vi "svx_Oct_Property Page.vi"(4 "# Plots Updated in":i32, 6 "Z Scale Graph Refnum":refnum<vi>, 7 "Main Graph":refnum<vi>, 8 "XY Scale Graph Refnum":refnum<vi>, 9 "Container Refnum":refnum<vi>, 10 "State in":T1={"X Scale Width %"=50.0, "Y Scale Height %"=50.0, "X-Axis Range"={"Minimum"=0.0, "Maximum"=10.0}, "Y-Axis Range"={"Minimum"=0.0, "Maximum"=10.0}, "Z-Axis Range"={"Minimum"=0.0, "Maximum"=10.0}, "Plot Color"=0, "Frame Color"=61212, "Background Color"=16252785, "Initial AutoScale Y"=TRUE, "AutoScale X"=2, "AutoScale Y"=2, "AutoScale Z"=2, "Plot Transparency"=FALSE, "X-Axis Name"="Frequency", "Y-Axis Name"="Amplitude", "Z-Axis Name"="", "X-Axis Scaling Factor"={"Offset"=0.0, "Multiplier"=1.0}, "Y-Axis Scaling Factor"={"Offset"=0.0, "Multiplier"=1.0}, "Z-Axis Scaling Factor"={"Offset"=0.0, "Multiplier"=1.0}, "X-Scale Visible"=TRUE, "Y-Scale Visible"=TRUE, "Z-Scale Visible"=TRUE, "X-Scale Label Visible"=TRUE, "Y-Scale Label Visible"=TRUE, "Z-Scale Label Visible"=TRUE, "X-Axis Range Scaled"={"Minimum"=0.0, "Maximum"=10.0}, "Y-Axis Range Scaled"={"Minimum"=0.0, "Maximum"=10.0}, "Z-Axis Range Scaled"={"Minimum"=0.0, "Maximum"=10.0}, "Rev Z Order"=FALSE, "X-Scale Format Str"="%#.4g", "Y-Scale Format Str"="%#.4g", "Z-Scale Format Str"="%#.4g", "Decor color"=12369084, "Scale Range Change"=refnum, "out of state queue"=refnum, "property nodes"=refnum} caption="State", 11 "Data In":T2={"z0"=0.0, "dz"=1.0, "Plots"=[]} {"Plots"."Y" format="%.2f"; "Plots"."X" format="%.2f"}) -> (0 "# Plots Updated out":i32, 1 "Cancel?":bool, 2 "State out":T1={"X Scale Width %"=50.0, "Y Scale Height %"=50.0, "X-Axis Range"={"Minimum"=0.0, "Maximum"=10.0}, "Y-Axis Range"={"Minimum"=0.0, "Maximum"=10.0}, "Z-Axis Range"={"Minimum"=0.0, "Maximum"=10.0}, "Plot Color"=0, "Frame Color"=61212, "Background Color"=16252785, "Initial AutoScale Y"=TRUE, "AutoScale X"=2, "AutoScale Y"=2, "AutoScale Z"=2, "Plot Transparency"=FALSE, "X-Axis Name"="Frequency", "Y-Axis Name"="Amplitude", "Z-Axis Name"="", "X-Axis Scaling Factor"={"Offset"=0.0, "Multiplier"=1.0}, "Y-Axis Scaling Factor"={"Offset"=0.0, "Multiplier"=1.0}, "Z-Axis Scaling Factor"={"Offset"=0.0, "Multiplier"=1.0}, "X-Scale Visible"=TRUE, "Y-Scale Visible"=TRUE, "Z-Scale Visible"=TRUE, "X-Scale Label Visible"=TRUE, "Y-Scale Label Visible"=TRUE, "Z-Scale Label Visible"=TRUE, "X-Axis Range Scaled"={"Minimum"=0.0, "Maximum"=10.0}, "Y-Axis Range Scaled"={"Minimum"=0.0, "Maximum"=10.0}, "Z-Axis Range Scaled"={"Minimum"=0.0, "Maximum"=10.0}, "Rev Z Order"=FALSE, "X-Scale Format Str"="%#.4g", "Y-Scale Format Str"="%#.4g", "Z-Scale Format Str"="%#.4g", "Decor color"=12369084, "Scale Range Change"=refnum, "out of state queue"=refnum, "property nodes"=refnum} caption="State")   [LabVIEW 2017, in "SVX Octave Waterfall Graph.xctl"]
uses:
  <vilib>/addons/_XControls/Octave Waterfall Graph/SVX Octave Waterfall Graph.xctl
  <vilib>/addons/_XControls/Octave Waterfall Graph/subVIs/svx_Oct_Waterfall Data.ctl
  <vilib>/addons/_XControls/Octave Waterfall Graph/subVIs/svx_Oct_Waterfall State.ctl
  <vilib>/addons/_XControls/Octave Waterfall Graph/subVIs/svx_Oct_Waterfall Property Page User Events.ctl
panel:
  in  "Help":bool
  in  "Cancel":bool
  in  "OK":bool
  in  "Tab Control":T3(tab)
  in  "Reverse Order":bool
  in  "Plot Transparency":bool
  in  "Background color":u32(colorbox)
  in  "Frame color":u32(colorbox)
  in  "Plot color":u32(colorbox)
  in  "Enable State":T4(radio)
  in  "Caption":string
  in  "Label":string
  in  "Caption Visible?":bool
  in  "Label Visible?":bool
  in  "trailing zeros":bool
  in  "Digits":u8=1
  in  "Precision Type":u16(ring) caption="Precision type" items=["Digits of precision", "Significant digits"]
  in  "Type":i32(listbox)
  in  "FP Axis":enum16{"X-Axis", "Y-Axis", "Z-Axis"}(ring)
  in  "Scaling Factors - Multiplier":dbl caption="Multiplier"
  in  "Scaling Factors - Offset":dbl caption="Offset"
  in  "Range Maximum":dbl caption="Maximum"
  in  "Range Minimum":dbl caption="Minimum"
  in  "Autoscale":bool
  in  "Show Scale":bool
  in  "Show Scale label":bool
  in  "Scale Name":string caption="Name"
  in  "Scale Axis":enum16{"X-Axis", "Y-Axis", "Z-Axis"}(ring)
  in  "Tip strip":string
  in  "Description":string
  # "Label"
  # "Caption"
  # "Enabled State"
  # "Color Scheme"
  # "Scaling factors"
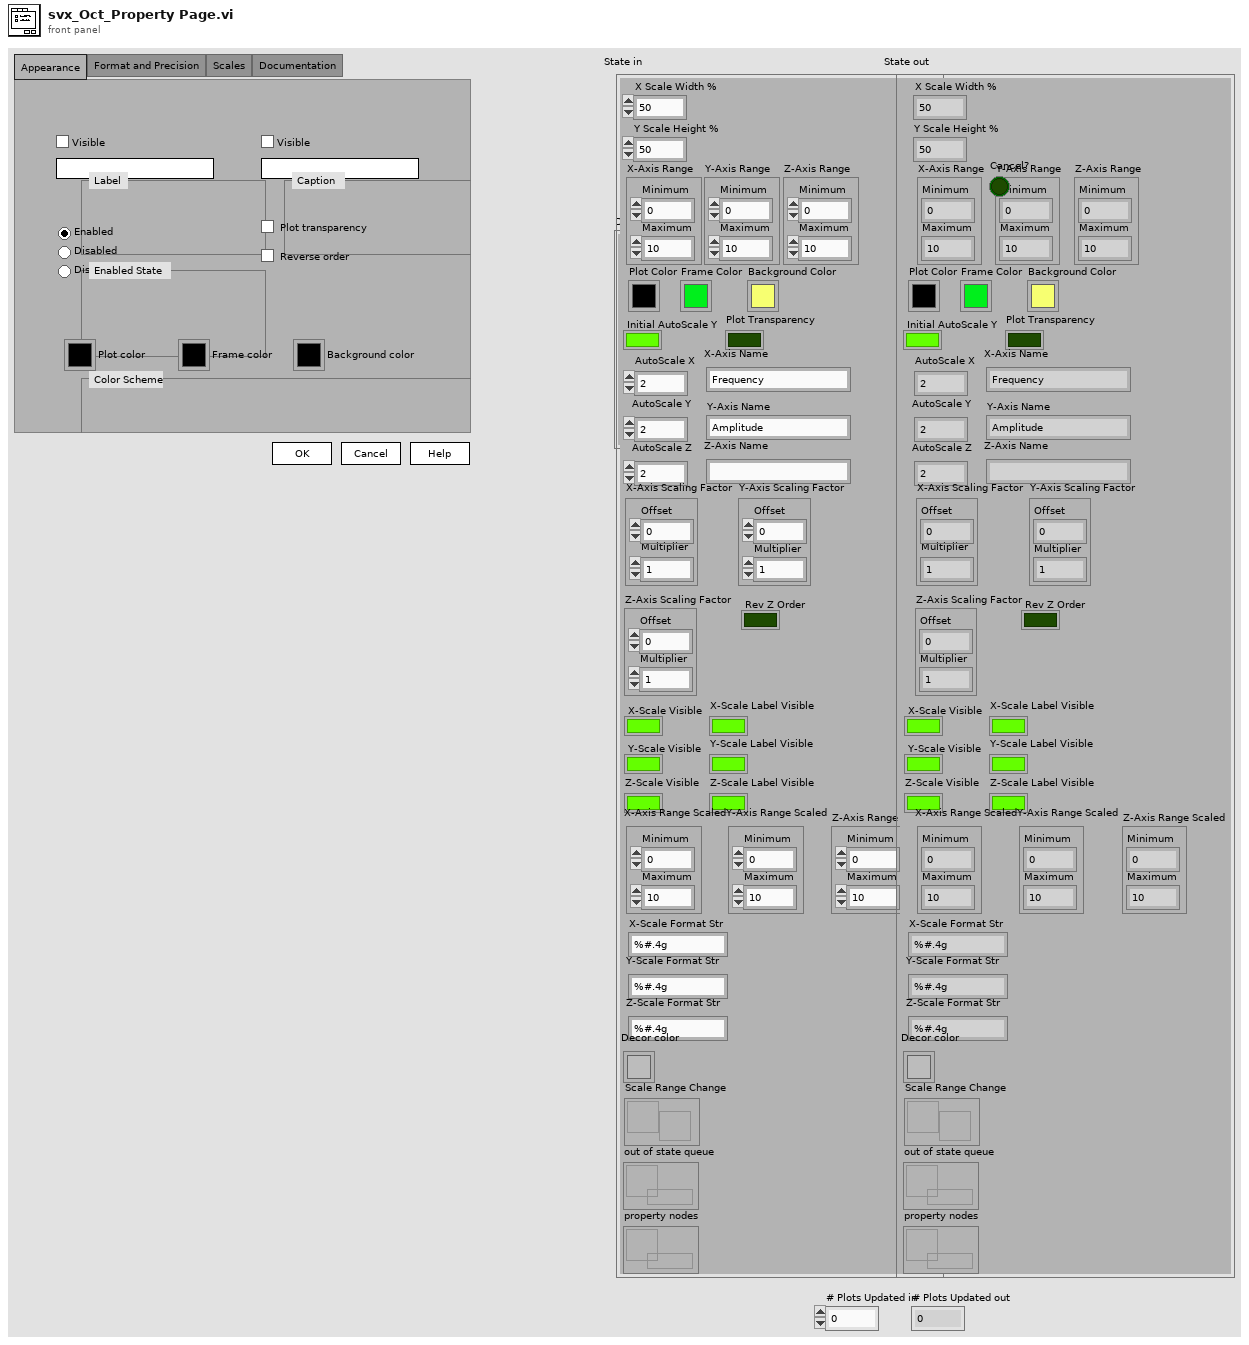
[diagram p1: front panel]
types:
  T1 = typedef "SVX Octave Waterfall Graph.xctl/svx_Oct_Waterfall State.ctl" = cluster{"X Scale Width %":dbl, "Y Scale Height %":dbl, "X-Axis Range":cluster{"Minimum":dbl, "Maximum":dbl}, "Y-Axis Range":cluster{"Minimum":dbl, "Maximum":dbl}, "Z-Axis Range":cluster{"Minimum":dbl, "Maximum":dbl}, "Plot Color":u32, "Frame Color":u32, "Background Color":u32, "Initial AutoScale Y":bool, "AutoScale X":u8, "AutoScale Y":u8, "AutoScale Z":u8, "Plot Transparency":bool, "X-Axis Name":string, "Y-Axis Name":string, "Z-Axis Name":string, "X-Axis Scaling Factor":cluster{"Offset":dbl, "Multiplier":dbl}, "Y-Axis Scaling Factor":cluster{"Offset":dbl, "Multiplier":dbl}, "Z-Axis Scaling Factor":cluster{"Offset":dbl, "Multiplier":dbl}, "X-Scale Visible":bool, "Y-Scale Visible":bool, "Z-Scale Visible":bool, "X-Scale Label Visible":bool, "Y-Scale Label Visible":bool, "Z-Scale Label Visible":bool, "X-Axis Range Scaled":cluster{"Minimum":dbl, "Maximum":dbl}, "Y-Axis Range Scaled":cluster{"Minimum":dbl, "Maximum":dbl}, "Z-Axis Range Scaled":cluster{"Minimum":dbl, "Maximum":dbl}, "Rev Z Order":bool, "X-Scale Format Str":string, "Y-Scale Format Str":string, "Z-Scale Format Str":string, "Decor color":u32, "Scale Range Change":refnum<user-event>, "out of state queue":refnum<queue>, "property nodes":refnum<queue>}
  T2 = typedef "SVX Octave Waterfall Graph.xctl/svx_Oct_Waterfall Data.ctl" = cluster{"z0":dbl, "dz":dbl, "Plots":cluster{"X":dbl[], "Y":dbl[]}[]}
  T3 = enum32{"Appearance", "Format and Precision", "Scales", "Documentation"}
  T4 = enum32{"Enabled", "Disabled", "Disabled & grayed"}
  T5 = typedef "SVX Octave Waterfall Graph.xctl/svx_Oct_Waterfall Property Page User Events.ctl" = enum16{"Redraw Frame", "Update Graph", "Exit"}
  T6 = cluster{"Container Changed":bool, "Scales Changed":bool, "Waveform Changed":bool}
  T7 = cluster{"Label.Text":string, "Label.Visible":bool, "Caption.Text":string, "Caption.Visible":bool, "Disabled":u8, "Desc":string, "TipStrip":string}
  T8 = cluster{"Width":u16, "Style":enum32{"Solid", "Dash", "Dot", "DashDot", "DashDotDot"}}
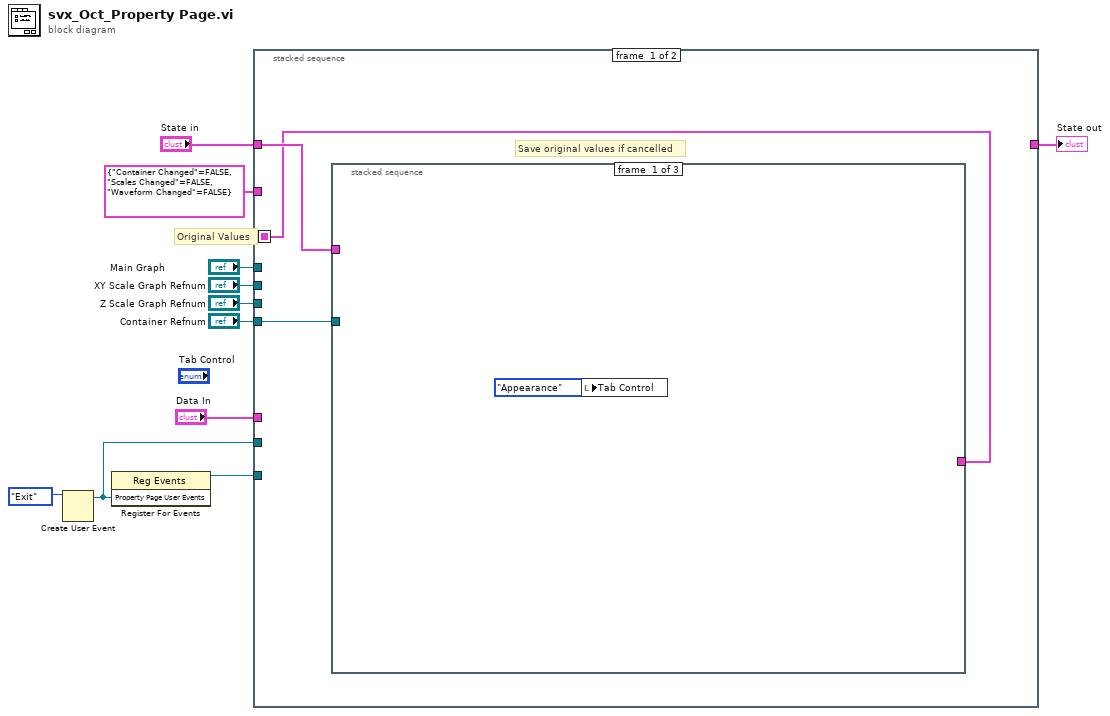
[diagram p0: block diagram]
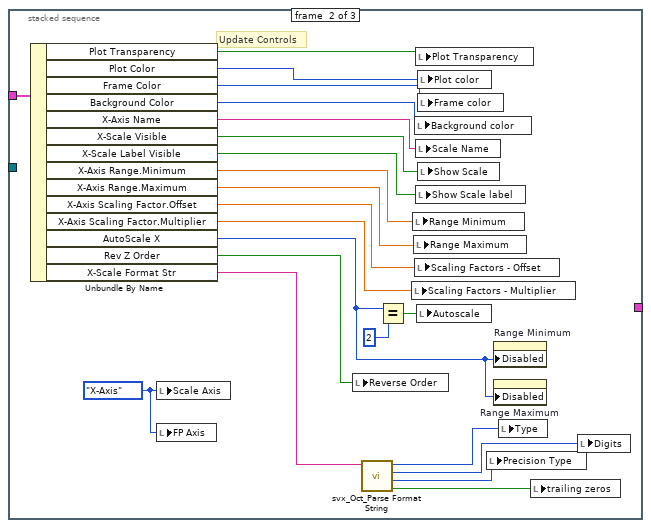
[diagram p2: hidden frame]
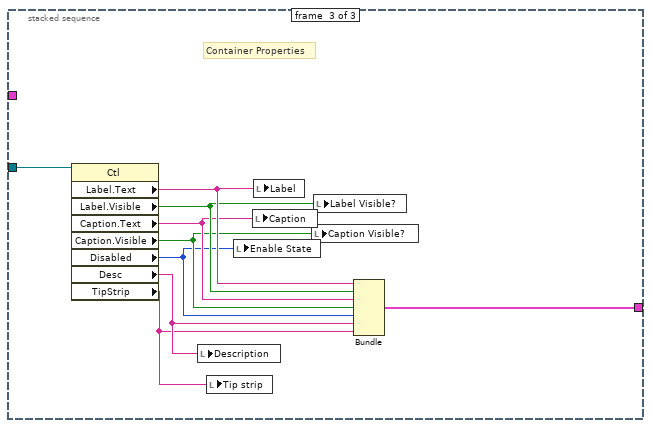
[diagram p3: hidden frame]
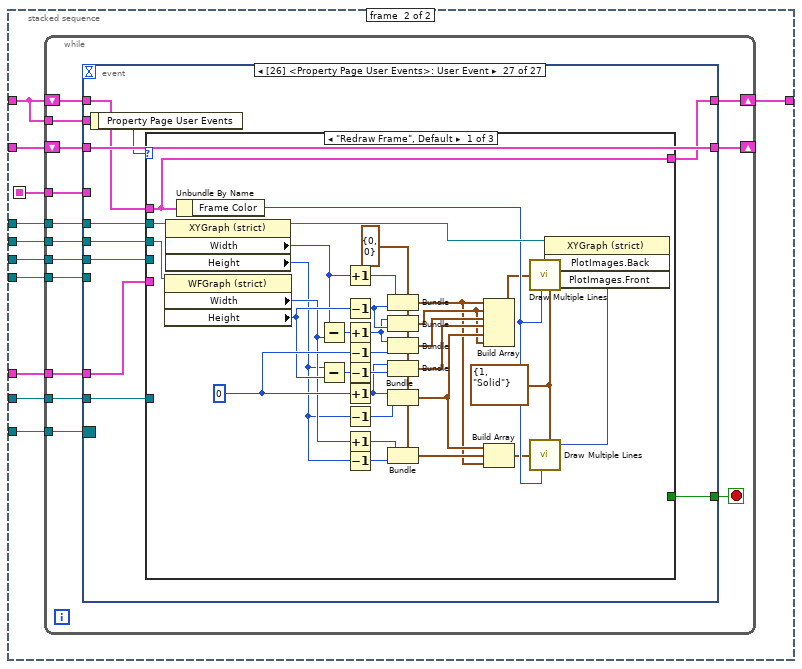
[diagram p4: hidden frame]
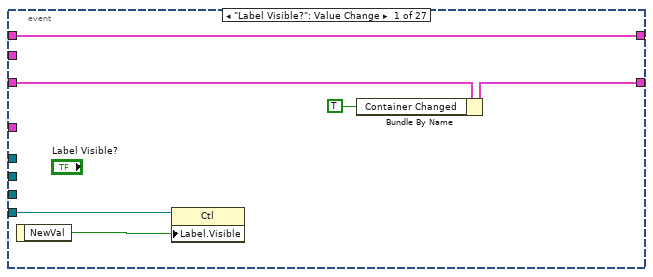
[diagram p5: hidden frame]
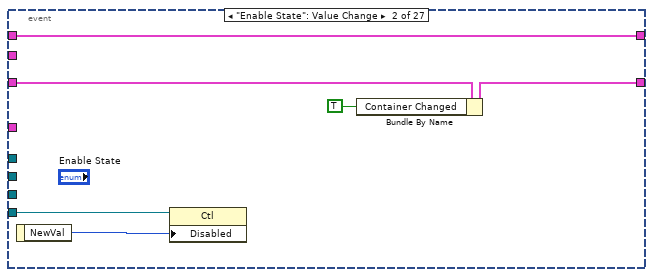
[diagram p6: hidden frame]
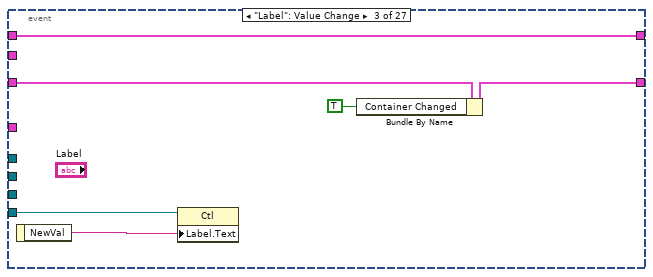
[diagram p7: hidden frame]
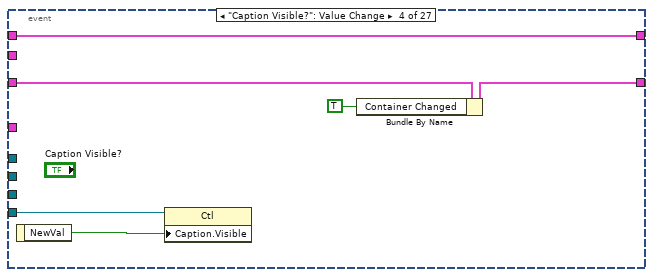
[diagram p8: hidden frame]
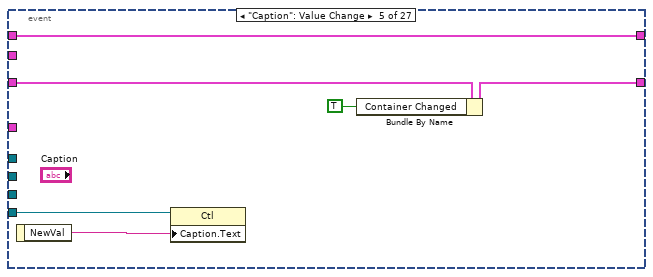
[diagram p9: hidden frame]
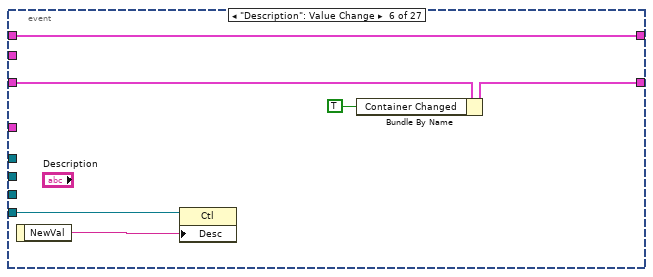
[diagram p10: hidden frame]
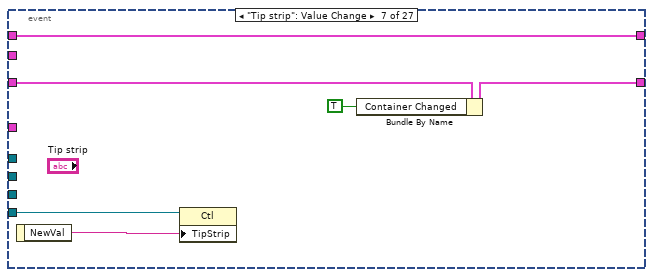
[diagram p11: hidden frame]
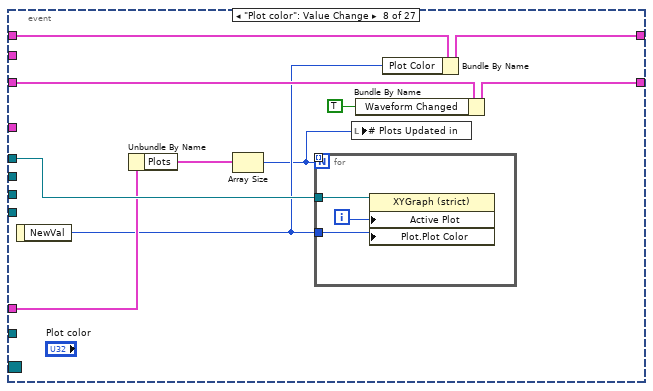
[diagram p12: hidden frame]
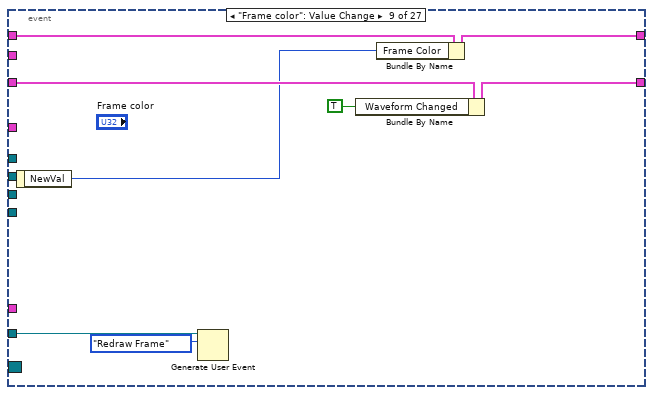
[diagram p13: hidden frame]
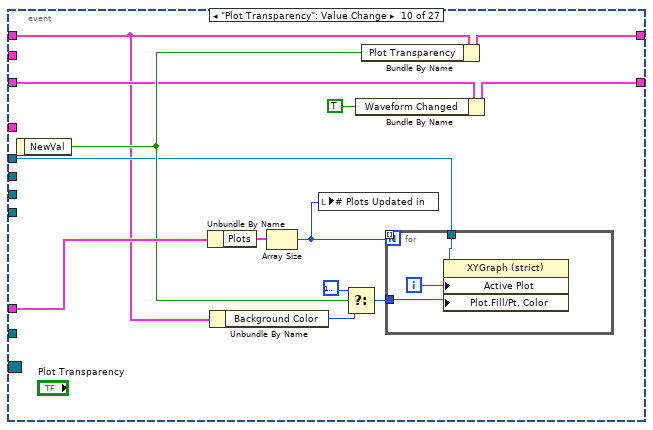
[diagram p14: hidden frame]
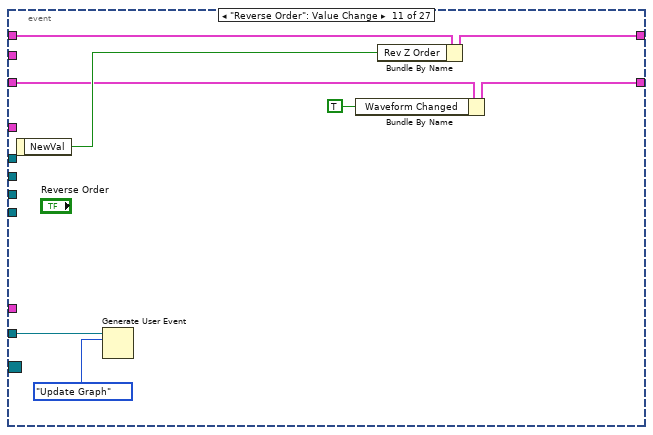
[diagram p15: hidden frame]
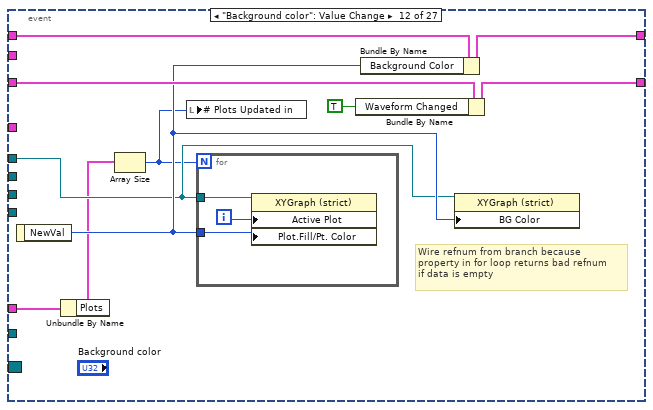
[diagram p16: hidden frame]
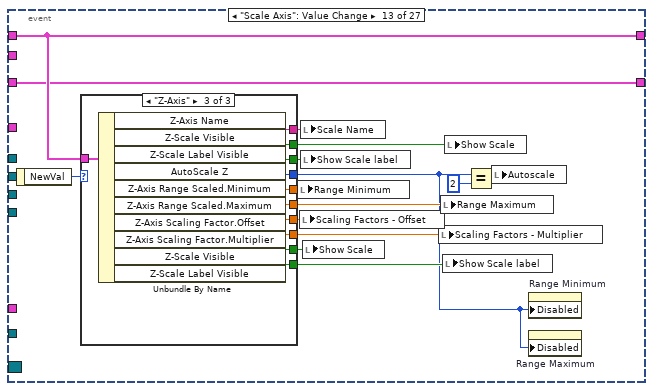
[diagram p17: hidden frame]
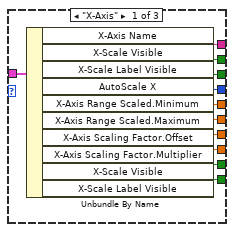
[diagram p18: hidden frame]
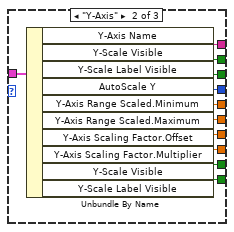
[diagram p19: hidden frame]
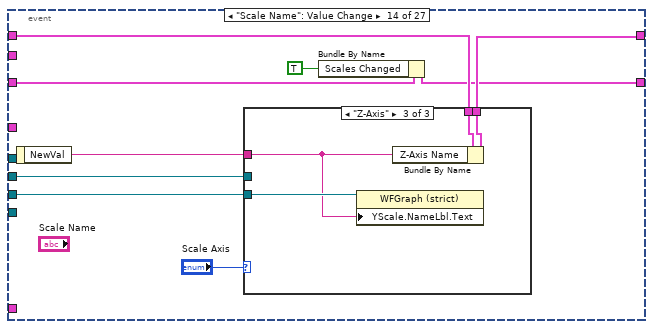
[diagram p20: hidden frame]
diagram:
  # "Original Values"
  n1 = Create User Event(user event datatype=svx_Oct_Waterfall_Property_Page_User_Events."Exit" ("Property Page User Events")) -> (user event=w1:refnum<user-event>)  [unwired: 1 in, 1 out]
  n2 = register-events(w1) -> (reference out=w3:refnum<event-registration>)  [unwired: 2 in, 1 out]
  n3 = stacked-sequence {
    seq-local: [w12 _] -> [_ w50]
    tunnel: T6 {"Container Changed"=FALSE, "Scales Changed"=FALSE, "Waveform Changed"=FALSE} -> [_ w57]
    tunnel: "Main Graph" -> [_ w56]
    tunnel: "XY Scale Graph Refnum" -> [_ w55]
    tunnel: "Z Scale Graph Refnum" -> [_ w54]
    tunnel: "Container Refnum" -> [w14 w53]
    tunnel: "State in" -> [w13 w51]
    tunnel: [_ w52] -> w5
    tunnel: "Data In" -> [_ w49]
    tunnel: w3 -> [_ w48]
    tunnel: w1 -> [_ w47]
    frame #0 {
      # "Save original values if cancelled"
      n4 = stacked-sequence {
        tunnel: w14 -> [_ _ w46]
        tunnel: [_ _ w45] -> w12
        tunnel: w13 -> [_ w37 _]
        frame #0 {
          n5 = local write "Tab Control"(T3."Appearance" ("Tab Control")) -> ()
        }
        frame #1 {
          w16 = enum16{"X-Axis", "Y-Axis", "Z-Axis"}."X-Axis" ("Axis")
          # "Update Controls"
          n6 = Unbundle By Name(w37) -> ("Plot Transparency"=w26:bool, "Plot Color"=w36:u32, "Frame Color"=w35:u32, "Background Color"=w34:u32, "X-Axis Name"=w33:string, "X-Scale Visible"=w32:bool, "X-Scale Label Visible"=w31:bool, "X-Axis Range.Minimum"=w30:dbl, "X-Axis Range.Maximum"=w29:dbl, "X-Axis Scaling Factor.Offset"=w28:dbl, "X-Axis Scaling Factor.Multiplier"=w27:dbl, "AutoScale X"=w25:u8, "Rev Z Order"=w22:bool, "X-Scale Format Str"=w21:string)
          n7 = local write "Scale Axis"(w16) -> ()
          n8 = local write "FP Axis"(w16) -> ()
          n9 = local write "Reverse Order"(w22) -> ()
          n10 = call <vilib>:"svx_Oct_Parse Format String.vi"("Format string"=w21) -> ("trailing zeros"=w17:bool, "Precision Type"=w18:u16, "Digits"=w19:u8, "Type"=w20:i32)  [unwired: 6 in, 1 out]
          n11 = Equal?(x=w25, y=u8 2) -> (x = y?=w23:bool)
          n12 = local write "Scaling Factors - Multiplier"(w27) -> ()
          n13 = local write "Range Minimum"(w30) -> ()
          n14 = local write "Range Maximum"(w29) -> ()
          n15 = local write "Background color"(w34) -> ()
          n16 = local write "Scaling Factors - Offset"(w28) -> ()
          n17 = local write "Plot Transparency"(w26) -> ()
          n18 = local write "Scale Name"(w33) -> ()
          n19 = local write "Show Scale label"(w31) -> ()
          n20 = local write "Autoscale"(w23) -> ()
          n21 = local write "Plot color"(w36) -> ()
          n22 = local write "Frame color"(w35) -> ()
          n23 = local write "Show Scale"(w32) -> ()
          n24 = local write "Precision Type"(w18) -> ()
          n25 = property on="Range Minimum" class="DigNum (strict)"("Disabled"=w25) -> ()  [unwired: 2 in, 2 out]
          n26 = property on="Range Maximum" class="DigNum (strict)"("Disabled"=w25) -> ()  [unwired: 2 in, 2 out]
          n27 = local write "Type"(w20) -> ()
          n28 = local write "trailing zeros"(w17) -> ()
          n29 = local write "Digits"(w19) -> ()
        }
        frame #2 {
          # "Container Properties"
          n30 = property class="Ctl"(reference=w46) -> ("Label.Text"=w44:string, "Label.Visible"=w43:bool, "Caption.Text"=w42:string, "Caption.Visible"=w41:bool, "Disabled"=w40:u8, "Desc"=w39:string, "TipStrip"=w38:string)  [unwired: 1 in, 2 out]
          n31 = local write "Description"(w39) -> ()
          n32 = local write "Tip strip"(w38) -> ()
          n33 = local write "Enable State"(w40) -> ()
          n34 = local write "Caption"(w42) -> ()
          n35 = local write "Label"(w44) -> ()
          n36 = local write "Caption Visible?"(w41) -> ()
          n37 = local write "Label Visible?"(w43) -> ()
          n38 = Bundle("Label.Text"=w44, "Label.Visible"=w43, "Caption.Text"=w42, "Caption.Visible"=w41, "Disabled"=w40, "Desc"=w39, "TipStrip"=w38) -> (w45:T7)  [unwired: 1 in]
        }
      }
    }
    frame #1 {
      n39 = while {
        shift-right: [w69] -> _
        shift-left: w57 -> [w70]
        tunnel: w56 -> [w68]
        tunnel: w55 -> [w67]
        tunnel: w54 -> [w66]
        tunnel: w53 -> [w65]
        shift-right: [w63] -> w52
        shift-left: w51 -> [w64]
        tunnel: w51 -> [w62]
        tunnel: w50 -> [w61]
        tunnel: w49 -> [w60]
        tunnel: w48 -> [w59]
        tunnel: w47 -> [w58]
        stop <- w71 stop-if-true
        n40 = event shown="[26] <Property Page User Events>: User Event" {
          selector: w59 -> [_ _ _ _ _ _ _ _ _ _ _ _ _ _ _ _ _ _ _ _ _ _ _ _ _ _ _]
          dyn-events: _ -> [_ _ _ _ _ _ _ _ _ _ _ _ _ _ _ _ _ _ _ _ _ _ _ _ _ _ _]
          timeout: _ -> [_ _ _ _ _ _ _ _ _ _ _ _ _ _ _ _ _ _ _ _ _ _ _ _ _ _ _]
          tunnel: [_ _ _ _ _ _ _ _ _ _ _ _ _ _ _ _ _ _ _ _ _ _ _ w547 _ _ w641] -> w71
          tunnel: w70 -> [w77 w83 w89 w95 w101 w107 w113 w123 w135 w141 w156 w170 w179 w223 w245 w266 w287 w338 w394 w442 w493 w514 w531 w551 w560 w630 w643]
          tunnel: [w76 w82 w88 w94 w100 w106 w112 w122 w134 w148 w160 w169 w179 w222 w244 w265 w286 w337 w393 w441 w492 w514 w530 w551 w560 w630 w643] -> w69
          tunnel: w68 -> [_ _ _ _ _ _ _ w120 _ w139 _ w163 _ _ _ _ _ _ w398 w446 _ _ _ _ w555 _ w640]
          tunnel: w67 -> [_ _ _ _ _ _ _ _ _ _ _ _ _ w226 w248 w269 w293 w344 w401 w449 _ _ w527 _ w553 _ w639]
          tunnel: w66 -> [_ _ _ _ _ _ _ _ _ _ _ _ _ w225 w247 w268 w292 w343 w400 w448 _ _ w526 _ w552 _ w635]
          tunnel: w65 -> [w74 w80 w86 w92 w98 w104 w110 _ _ _ _ _ _ _ _ _ _ _ _ _ _ _ _ _ w559 _ _]
          tunnel: w64 -> [w72 w78 w84 w90 w96 w102 w108 w119 w132 w138 w155 w167 w187 w230 w251 w272 w296 w347 w404 w452 w498 w513 w534 w550 _ w629 w637]
          tunnel: [w72 w78 w84 w90 w96 w102 w108 w118 w131 w146 w158 w166 w187 w229 w250 w271 w295 w346 w403 w451 w497 w513 w533 w550 w557 w629 w634] -> w63
          tunnel: w62 -> [_ _ _ _ _ _ _ _ _ _ _ _ _ _ _ _ _ _ _ _ _ _ _ _ w557 _ _]
          tunnel: w61 -> [_ _ _ _ _ _ _ _ _ _ _ _ _ _ _ _ _ _ _ _ _ _ _ _ w554 _ _]
          tunnel: w60 -> [_ _ _ _ _ _ _ w117 _ w144 _ w165 _ _ _ _ _ _ _ _ _ _ _ _ w556 _ w638]
          tunnel: w58 -> [_ _ _ _ _ _ _ _ w129 _ w153 _ _ _ _ _ w285 w336 w397 w445 w496 _ _ w548 w558 _ w636]
          event "Label Visible?": Value Change {
            n41 = event-data() -> ("NewVal"=w73:bool)  [unwired: 1 in]
            n42 = property class="Ctl"(reference=w74, "Label.Visible"=w73) -> ()  [unwired: 1 in, 2 out]
            n43 = Bundle By Name(cluster=w77, "Container Changed"=TRUE) -> (w76:T6)
          }
          event "Enable State": Value Change {
            n44 = event-data() -> ("NewVal"=w79:T4)  [unwired: 1 in]
            n45 = property class="Ctl"(reference=w80, "Disabled"=w79) -> ()  [unwired: 1 in, 2 out]
            n46 = Bundle By Name(cluster=w83, "Container Changed"=TRUE) -> (w82:T6)
          }
          event "Label": Value Change {
            n47 = event-data() -> ("NewVal"=w85:string)  [unwired: 1 in]
            n48 = property class="Ctl"(reference=w86, "Label.Text"=w85) -> ()  [unwired: 1 in, 2 out]
            n49 = Bundle By Name(cluster=w89, "Container Changed"=TRUE) -> (w88:T6)
          }
          event "Caption Visible?": Value Change {
            n50 = event-data() -> ("NewVal"=w91:bool)  [unwired: 1 in]
            n51 = property class="Ctl"(reference=w92, "Caption.Visible"=w91) -> ()  [unwired: 1 in, 2 out]
            n52 = Bundle By Name(cluster=w95, "Container Changed"=TRUE) -> (w94:T6)
          }
          event "Caption": Value Change {
            n53 = event-data() -> ("NewVal"=w97:string)  [unwired: 1 in]
            n54 = property class="Ctl"(reference=w98, "Caption.Text"=w97) -> ()  [unwired: 1 in, 2 out]
            n55 = Bundle By Name(cluster=w101, "Container Changed"=TRUE) -> (w100:T6)
          }
          event "Description": Value Change {
            n56 = event-data() -> ("NewVal"=w103:string)  [unwired: 1 in]
            n57 = property class="Ctl"(reference=w104, "Desc"=w103) -> ()  [unwired: 1 in, 2 out]
            n58 = Bundle By Name(cluster=w107, "Container Changed"=TRUE) -> (w106:T6)
          }
          event "Tip strip": Value Change {
            n59 = event-data() -> ("NewVal"=w109:string)  [unwired: 1 in]
            n60 = property class="Ctl"(reference=w110, "TipStrip"=w109) -> ()  [unwired: 1 in, 2 out]
            n61 = Bundle By Name(cluster=w113, "Container Changed"=TRUE) -> (w112:T6)
          }
          event "Plot color": Value Change {
            n62 = event-data() -> ("NewVal"=w116:u32)  [unwired: 1 in]
            n63 = Unbundle By Name(w117) -> ("Plots"=w115:cluster{"X":dbl[], "Y":dbl[]}[])
            n64 = Array Size(array=w115) -> (size(s)=w114:i32)
            n65 = for {
              N: w114 -> [w124]
              tunnel: w116 -> [w126]
              tunnel: w120 -> [w127]
              tunnel: [w124] -> _ mode=indexing
              i -> [w125]
              n66 = property class="XYGraph (strict)"(reference=w127, "Active Plot"=w125, "Plot.Plot Color"=w126) -> ()  [unwired: 1 in, 2 out]
            }
            n67 = local write "# Plots Updated in"(w114) -> ()
            n68 = Bundle By Name(cluster=w123, "Waveform Changed"=TRUE ("Container Changed")) -> (w122:T6)
            n69 = Bundle By Name(cluster=w119, "Plot Color"=w116) -> (w118:T1)
          }
          event "Frame color": Value Change {
            n70 = event-data() -> ("NewVal"=w130:u32)  [unwired: 1 in]
            n71 = Generate User Event(user event=w129, event data cluster=svx_Oct_Waterfall_Property_Page_User_Events."Redraw Frame" ("Property Page User Events")) -> ()  [unwired: 2 in, 2 out]
            n72 = Bundle By Name(cluster=w135, "Waveform Changed"=TRUE ("Container Changed")) -> (w134:T6)
            n73 = Bundle By Name(cluster=w132, "Frame Color"=w130) -> (w131:T1)
          }
          event "Plot Transparency": Value Change {
            n74 = event-data() -> ("NewVal"=w143:bool)  [unwired: 1 in]
            n75 = Unbundle By Name(w144) -> ("Plots"=w137:cluster{"X":dbl[], "Y":dbl[]}[])
            n76 = Unbundle By Name(w138) -> ("Background Color"=w140:u32)
            n77 = Array Size(array=w137) -> (size(s)=w136:i32)
            n78 = local write "# Plots Updated in"(w136) -> ()
            n79 = Select(t=u32 16777216, s=w143, f=w140) -> (s? t:f=w145:u32)
            n80 = Bundle By Name(cluster=w141, "Waveform Changed"=TRUE) -> (w148:T6)
            n81 = Bundle By Name(cluster=w138, "Plot Transparency"=w143) -> (w146:T1)
            n82 = for {
              N: w136 -> [w149]
              tunnel: w145 -> [w151]
              tunnel: w139 -> [w150]
              tunnel: [w149] -> _ mode=indexing
              i -> [w152]
              n83 = property on="Property Node" class="XYGraph (strict)"(reference=w150, "Active Plot"=w152, "Plot.Fill/Pt. Color"=w151) -> ()  [unwired: 1 in, 2 out]
            }
          }
          event "Reverse Order": Value Change {
            n84 = event-data() -> ("NewVal"=w157:bool)  [unwired: 1 in]
            n85 = Generate User Event(user event=w153, event data cluster=svx_Oct_Waterfall_Property_Page_User_Events."Update Graph" ("event data")) -> ()  [unwired: 2 in, 2 out]
            n86 = Bundle By Name(cluster=w156, "Waveform Changed"=TRUE) -> (w160:T6)
            n87 = Bundle By Name(cluster=w155, "Rev Z Order"=w157) -> (w158:T1)
          }
          event "Background color": Value Change {
            # "Wire refnum from branch because\nproperty in for loop returns bad refnum\nif data is empty"
            n88 = event-data() -> ("NewVal"=w164:u32)  [unwired: 1 in]
            n89 = Unbundle By Name(w165) -> ("Plots"=w162:cluster{"X":dbl[], "Y":dbl[]}[])
            n90 = Array Size(array=w162) -> (size(s)=w161:i32)
            n91 = local write "# Plots Updated in"(w161) -> ()
            n92 = for {
              N: w161 -> [_]
              tunnel: w164 -> [w172]
              tunnel: w163 -> [w173]
              i -> [w171]
              n93 = property class="XYGraph (strict)"(reference=w173, "Active Plot"=w171, "Plot.Fill/Pt. Color"=w172) -> ()  [unwired: 1 in, 2 out]
            }
            n94 = Bundle By Name(cluster=w170, "Waveform Changed"=TRUE ("Container Changed")) -> (w169:T6)
            n95 = Bundle By Name(cluster=w167, "Background Color"=w164) -> (w166:T1)
            n96 = property class="XYGraph (strict)"(reference=w163, "BG Color"=w164) -> ()  [unwired: 1 in, 2 out]
          }
          event "Scale Axis": Value Change {
            n97 = event-data() -> ("NewVal"=w188:enum16{"X-Axis", "Y-Axis", "Z-Axis"})  [unwired: 1 in]
            n98 = case shown="\"Z-Axis\"" w188 {
              tunnel: w187 -> [w199 w210 w221]
              tunnel: [w198 w209 w220] -> w176
              tunnel: [w197 w208 w219] -> w186
              tunnel: [w196 w207 w218] -> w185
              tunnel: [w195 w206 w217] -> w184
              tunnel: [w194 w205 w216] -> w183
              tunnel: [w193 w204 w215] -> w182
              tunnel: [w192 w203 w214] -> w181
              tunnel: [w191 w202 w213] -> w180
              tunnel: [w190 w201 w212] -> w178
              tunnel: [w189 w200 w211] -> w177
              frame "X-Axis" {
                n99 = Unbundle By Name(w199) -> ("X-Axis Name"=w191:string, "X-Scale Visible"=w192:bool, "X-Scale Label Visible"=w193:bool, "AutoScale X"=w198:u8, "X-Axis Range Scaled.Minimum"=w197:dbl, "X-Axis Range Scaled.Maximum"=w196:dbl, "X-Axis Scaling Factor.Offset"=w195:dbl, "X-Axis Scaling Factor.Multiplier"=w194:dbl, "X-Scale Visible"=w190:bool, "X-Scale Label Visible"=w189:bool)
              }
              frame "Y-Axis" {
                n100 = Unbundle By Name(w210) -> ("Y-Axis Name"=w202:string, "Y-Scale Visible"=w203:bool, "Y-Scale Label Visible"=w204:bool, "AutoScale Y"=w209:u8, "Y-Axis Range Scaled.Minimum"=w208:dbl, "Y-Axis Range Scaled.Maximum"=w207:dbl, "Y-Axis Scaling Factor.Offset"=w206:dbl, "Y-Axis Scaling Factor.Multiplier"=w205:dbl, "Y-Scale Visible"=w201:bool, "Y-Scale Label Visible"=w200:bool)
              }
              frame "Z-Axis" {
                n101 = Unbundle By Name(w221) -> ("Z-Axis Name"=w213:string, "Z-Scale Visible"=w214:bool, "Z-Scale Label Visible"=w215:bool, "AutoScale Z"=w220:u8, "Z-Axis Range Scaled.Minimum"=w219:dbl, "Z-Axis Range Scaled.Maximum"=w218:dbl, "Z-Axis Scaling Factor.Offset"=w217:dbl, "Z-Axis Scaling Factor.Multiplier"=w216:dbl, "Z-Scale Visible"=w212:bool, "Z-Scale Label Visible"=w211:bool)
              }
            }
            n102 = local write "Range Minimum"(w186) -> ()
            n103 = local write "Scaling Factors - Offset"(w184) -> ()
            n104 = local write "Scale Name"(w180) -> ()
            n105 = local write "Show Scale label"(w182) -> ()
            n106 = local write "Show Scale"(w178) -> ()
            n107 = local write "Scaling Factors - Multiplier"(w183) -> ()
            n108 = local write "Range Maximum"(w185) -> ()
            n109 = local write "Show Scale label"(w177) -> ()
            n110 = local write "Show Scale"(w181) -> ()
            n111 = Equal?(x=w176, y=u8 2) -> (x = y?=w174:bool)
            n112 = local write "Autoscale"(w174) -> ()
            n113 = property on="Range Minimum" class="DigNum (strict)"("Disabled"=w176) -> ()  [unwired: 2 in, 2 out]
            n114 = property on="Range Maximum" class="DigNum (strict)"("Disabled"=w176) -> ()  [unwired: 2 in, 2 out]
          }
          event "Scale Name": Value Change {
            n115 = event-data() -> ("NewVal"=w227:string)  [unwired: 1 in]
            n116 = case shown="\"Z-Axis\"" "Scale Axis" {
              tunnel: w230 -> [w234 w238 w242]
              tunnel: [w233 w237 w241] -> w229
              tunnel: w227 -> [w232 w235 w239]
              tunnel: w226 -> [w231 w236 _]
              tunnel: w225 -> [_ _ w240]
              frame "X-Axis" {
                n117 = property class="WFGraph (strict)"(reference=w231, "XScale.NameLbl.Text"=w232) -> ()  [unwired: 1 in, 2 out]
                n118 = Bundle By Name(cluster=w234, "X-Axis Name"=w232) -> (w233:T1)
              }
              frame "Y-Axis" {
                n119 = property class="WFGraph (strict)"(reference=w236, "YScale.NameLbl.Text"=w235) -> ()  [unwired: 1 in, 2 out]
                n120 = Bundle By Name(cluster=w238, "Y-Axis Name"=w235) -> (w237:T1)
              }
              frame "Z-Axis" {
                n121 = property class="WFGraph (strict)"(reference=w240, "YScale.NameLbl.Text"=w239) -> ()  [unwired: 1 in, 2 out]
                n122 = Bundle By Name(cluster=w242, "Z-Axis Name"=w239) -> (w241:T1)
              }
            }
            n123 = Bundle By Name(cluster=w223, "Scales Changed"=TRUE) -> (w222:T6)
          }
          event "Show Scale": Value Change {
            n124 = event-data() -> ("NewVal"=w249:bool)  [unwired: 1 in]
            n125 = local read "Scale Axis"() -> (w243:enum16{"X-Axis", "Y-Axis", "Z-Axis"})
            n126 = case shown="\"Y-Axis\"" w243 {
              tunnel: w251 -> [w255 w259 w263]
              tunnel: [w254 w258 w262] -> w250
              tunnel: w249 -> [w253 w256 w260]
              tunnel: w248 -> [w252 w257 _]
              tunnel: w247 -> [_ _ w261]
              frame "X-Axis" {
                n127 = property class="WFGraph (strict)"(reference=w252, "XScale.Visible"=w253) -> ()  [unwired: 1 in, 2 out]
                n128 = Bundle By Name(cluster=w255, "X-Scale Visible"=w253) -> (w254:T1)
              }
              frame "Y-Axis" {
                n129 = property class="WFGraph (strict)"(reference=w257, "YScale.Visible"=w256) -> ()  [unwired: 1 in, 2 out]
                n130 = Bundle By Name(cluster=w259, "Y-Scale Visible"=w256) -> (w258:T1)
              }
              frame "Z-Axis" {
                n131 = property class="WFGraph (strict)"(reference=w261, "YScale.Visible"=w260) -> ()  [unwired: 1 in, 2 out]
                n132 = Bundle By Name(cluster=w263, "Z-Scale Visible"=w260) -> (w262:T1)
              }
            }
            n133 = Bundle By Name(cluster=w245, "Scales Changed"=TRUE) -> (w244:T6)
          }
          event "Show Scale label": Value Change {
            n134 = event-data() -> ("NewVal"=w270:bool)  [unwired: 1 in]
            n135 = local read "Scale Axis"() -> (w264:enum16{"X-Axis", "Y-Axis", "Z-Axis"})
            n136 = case shown="\"Y-Axis\"" w264 {
              tunnel: w272 -> [w276 w280 w284]
              tunnel: [w275 w279 w283] -> w271
              tunnel: w270 -> [w274 w277 w281]
              tunnel: w269 -> [w273 w278 _]
              tunnel: w268 -> [_ _ w282]
              frame "X-Axis" {
                n137 = Bundle By Name(cluster=w276, "X-Scale Label Visible"=w274) -> (w275:T1)
                n138 = property class="WFGraph (strict)"(reference=w273, "XScale.NameLbl.Visible"=w274) -> ()  [unwired: 1 in, 2 out]
              }
              frame "Y-Axis" {
                n139 = Bundle By Name(cluster=w280, "Y-Scale Label Visible"=w277) -> (w279:T1)
                n140 = property class="WFGraph (strict)"(reference=w278, "YScale.NameLbl.Visible"=w277) -> ()  [unwired: 1 in, 2 out]
              }
              frame "Z-Axis" {
                n141 = Bundle By Name(cluster=w284, "Z-Scale Label Visible"=w281) -> (w283:T1)
                n142 = property class="WFGraph (strict)"(reference=w282, "YScale.NameLbl.Visible"=w281) -> ()  [unwired: 1 in, 2 out]
              }
            }
            n143 = Bundle By Name(cluster=w266, "Scales Changed"=TRUE) -> (w265:T6)
          }
          event "Scaling Factors - Offset": Value Change {
            n144 = local read "Scale Axis"() -> (w291:enum16{"X-Axis", "Y-Axis", "Z-Axis"})
            n145 = event-data() -> ("NewVal"=w294:dbl)  [unwired: 1 in]
            n146 = case shown="\"Z-Axis\"" w291 {
              tunnel: w296 -> [w306 w319 w334]
              tunnel: [w307 w320 w335] -> w295
              tunnel: w294 -> [w300 w313 w328]
              tunnel: w293 -> [w297 w312 _]
              tunnel: w292 -> [_ _ w327]
              tunnel: [w299 w309 w323] -> w290
              tunnel: [w298 w308 w322] -> w289
              tunnel: w285 -> [_ _ w325]
              frame "X-Axis" {
                n147 = Unbundle By Name(w306) -> ("X-Axis Range.Minimum"=w305:dbl, "X-Axis Scaling Factor.Multiplier"=w302:dbl, "X-Axis Range.Maximum"=w303:dbl)
                n148 = Multiply(x=w305, y=w302) -> (x*y=w304:dbl)
                n149 = Multiply(x=w302, y=w303) -> (x*y=w301:dbl)
                n150 = Add(x=w300, y=w304) -> (x+y=w299:dbl)
                n151 = Add(x=w300, y=w301) -> (x+y=w298:dbl)
                n152 = Bundle By Name(cluster=w306, "X-Axis Scaling Factor.Offset"=w300, "X-Axis Range Scaled.Minimum"=w299, "X-Axis Range Scaled.Maximum"=w298) -> (w307:T1)
                n153 = property class="WFGraph (strict)"(reference=w297, "XScale.Minimum"=w299, "XScale.Maximum"=w298) -> ()  [unwired: 1 in, 2 out]
              }
              frame "Y-Axis" {
                n154 = Unbundle By Name(w319) -> ("Y-Axis Range.Minimum"=w318:dbl, "Y-Axis Scaling Factor.Multiplier"=w315:dbl, "Y-Axis Range.Maximum"=w316:dbl)
                n155 = Multiply(x=w318, y=w315) -> (x*y=w317:dbl)
                n156 = Multiply(x=w315, y=w316) -> (x*y=w314:dbl)
                n157 = Add(x=w313, y=w317) -> (x+y=w311:dbl)
                n158 = Add(x=w313, y=w314) -> (x+y=w310:dbl)
                n159 = Max & Min(x=w311, y=w310) -> (max(x,y)=w308:dbl, min(x,y)=w309:dbl)
                n160 = Bundle By Name(cluster=w319, "Y-Axis Scaling Factor.Offset"=w313, "Y-Axis Range Scaled.Minimum"=w309, "Y-Axis Range Scaled.Maximum"=w308) -> (w320:T1)
                n161 = property class="WFGraph (strict)"(reference=w312, "YScale.Minimum"=w309, "YScale.Maximum"=w308) -> ()  [unwired: 1 in, 2 out]
              }
              frame "Z-Axis" {
                # "Needed to update\nZ-axis markers"
                n162 = Unbundle By Name(w334) -> ("Z-Axis Range.Minimum"=w333:dbl, "Z-Axis Scaling Factor.Multiplier"=w330:dbl, "Z-Axis Range.Maximum"=w331:dbl)
                n163 = Generate User Event(user event=w325, event data cluster=svx_Oct_Waterfall_Property_Page_User_Events."Update Graph" ("event data")) -> ()  [unwired: 2 in, 2 out]
                n164 = Multiply(x=w333, y=w330) -> (x*y=w332:dbl)
                n165 = Multiply(x=w330, y=w331) -> (x*y=w329:dbl)
                n166 = Add(x=w328, y=w332) -> (x+y=w324:dbl)
                n167 = Add(x=w328, y=w329) -> (x+y=w321:dbl)
                n168 = Max & Min(x=w324, y=w321) -> (max(x,y)=w322:dbl, min(x,y)=w323:dbl)
                n169 = Bundle By Name(cluster=w334, "Z-Axis Scaling Factor.Offset"=w328, "Z-Axis Range Scaled.Minimum"=w323, "Z-Axis Range Scaled.Maximum"=w322) -> (w335:T1)
                n170 = property class="WFGraph (strict)"(reference=w327, "YScale.Minimum"=w323, "YScale.Maximum"=w322) -> ()  [unwired: 1 in, 2 out]
              }
            }
            n171 = Bundle By Name(cluster=w287, "Scales Changed"=TRUE) -> (w286:T6)
            n172 = local write "Range Minimum"(w290) -> ()
            n173 = local write "Range Maximum"(w289) -> ()
          }
          event "Scaling Factors - Multiplier": Value Change {
            n174 = event-data() -> ("NewVal"=w345:dbl)  [unwired: 1 in]
            n175 = local read "Scale Axis"() -> (w342:enum16{"X-Axis", "Y-Axis", "Z-Axis"})
            n176 = case shown="\"Z-Axis\"" w342 {
              tunnel: w347 -> [w360 w374 w389]
              tunnel: [w361 w375 w390] -> w346
              tunnel: w345 -> [w352 w367 w383]
              tunnel: w344 -> [w354 w369 _]
              tunnel: w343 -> [_ _ w384]
              tunnel: [w349 w362 w376] -> w341
              tunnel: [w348 w363 w377] -> w340
              tunnel: w336 -> [_ _ w380]
              frame "X-Axis" {
                n177 = Unbundle By Name(w360) -> ("X-Axis Range.Minimum"=w359:dbl, "X-Axis Scaling Factor.Offset"=w355:dbl, "X-Axis Range.Maximum"=w357:dbl)
                n178 = Multiply(x=w352, y=w359) -> (x*y=w358:dbl)
                n179 = Multiply(x=w352, y=w357) -> (x*y=w356:dbl)
                n180 = Add(x=w358, y=w355) -> (x+y=w350:dbl)
                n181 = Add(x=w355, y=w356) -> (x+y=w351:dbl)
                n182 = Max & Min(x=w350, y=w351) -> (max(x,y)=w348:dbl, min(x,y)=w349:dbl)
                n183 = Bundle By Name(cluster=w360, "X-Axis Scaling Factor.Multiplier"=w352, "X-Axis Range Scaled.Maximum"=w348, "X-Axis Range Scaled.Minimum"=w349) -> (w361:T1)
                n184 = Less Than 0?(x=w352) -> (x < 0?=w353:bool)
                n185 = property class="WFGraph (strict)"(reference=w354, "XScale.Flipped"=w353, "XScale.Maximum"=w348, "XScale.Minimum"=w349) -> ()  [unwired: 1 in, 2 out]
              }
              frame "Y-Axis" {
                n186 = Unbundle By Name(w374) -> ("Y-Axis Range.Minimum"=w373:dbl, "Y-Axis Scaling Factor.Offset"=w368:dbl, "Y-Axis Range.Maximum"=w371:dbl)
                n187 = Multiply(x=w367, y=w373) -> (x*y=w372:dbl)
                n188 = Multiply(x=w367, y=w371) -> (x*y=w370:dbl)
                n189 = Add(x=w372, y=w368) -> (x+y=w365:dbl)
                n190 = Add(x=w368, y=w370) -> (x+y=w364:dbl)
                n191 = Max & Min(x=w365, y=w364) -> (max(x,y)=w363:dbl, min(x,y)=w362:dbl)
                n192 = Bundle By Name(cluster=w374, "Y-Axis Scaling Factor.Multiplier"=w367, "Y-Axis Range Scaled.Maximum"=w363, "Y-Axis Range Scaled.Minimum"=w362) -> (w375:T1)
                n193 = Less Than 0?(x=w367) -> (x < 0?=w366:bool)
                n194 = property class="WFGraph (strict)"(reference=w369, "YScale.Flipped"=w366, "YScale.Maximum"=w363, "YScale.Minimum"=w362) -> ()  [unwired: 1 in, 2 out]
              }
              frame "Z-Axis" {
                # "Needed to update\nZ-axis markers"
                n195 = Unbundle By Name(w389) -> ("Z-Axis Range.Minimum"=w388:dbl, "Z-Axis Scaling Factor.Offset"=w382:dbl, "Z-Axis Range.Maximum"=w386:dbl)
                n196 = Generate User Event(user event=w380, event data cluster=svx_Oct_Waterfall_Property_Page_User_Events."Update Graph" ("event data")) -> ()  [unwired: 2 in, 2 out]
                n197 = Multiply(x=w383, y=w388) -> (x*y=w387:dbl)
                n198 = Multiply(x=w383, y=w386) -> (x*y=w385:dbl)
                n199 = Add(x=w387, y=w382) -> (x+y=w379:dbl)
                n200 = Add(x=w382, y=w385) -> (x+y=w378:dbl)
                n201 = Max & Min(x=w379, y=w378) -> (max(x,y)=w377:dbl, min(x,y)=w376:dbl)
                n202 = Bundle By Name(cluster=w389, "Z-Axis Scaling Factor.Multiplier"=w383, "Z-Axis Range Scaled.Minimum"=w376, "Z-Axis Range Scaled.Maximum"=w377) -> (w390:T1)
                n203 = property class="WFGraph (strict)"(reference=w384, "YScale.Minimum"=w376, "YScale.Maximum"=w377) -> ()  [unwired: 1 in, 2 out]
              }
            }
            n204 = Bundle By Name(cluster=w338, "Scales Changed"=TRUE) -> (w337:T6)
            n205 = local write "Range Minimum"(w341) -> ()
            n206 = local write "Range Maximum"(w340) -> ()
          }
          event "Range Minimum": Value Change {
            n207 = event-data() -> ("NewVal"=w402:dbl)  [unwired: 1 in]
            n208 = local read "Scale Axis"() -> (w399:enum16{"X-Axis", "Y-Axis", "Z-Axis"})
            n209 = Generate User Event(user event=w397, event data cluster=svx_Oct_Waterfall_Property_Page_User_Events."Update Graph" ("event data")) -> ()  [unwired: 2 in, 2 out]
            n210 = case shown="\"Z-Axis\"" w399 {
              tunnel: w404 -> [w415 w427 w437]
              tunnel: [w416 w428 w438] -> w403
              tunnel: w402 -> [w409 w417 w432]
              tunnel: w401 -> [w414 w426 _]
              tunnel: w400 -> [_ _ _]
              tunnel: w398 -> [_ _ _]
              tunnel: [w408 w424 w436] -> w392
              tunnel: [w407 w425 w434] -> w391
              frame "X-Axis" {
                n211 = Unbundle By Name(w415) -> ("X-Axis Range Scaled.Maximum"=w410:dbl, "X-Axis Scaling Factor.Multiplier"=w412:dbl, "X-Axis Scaling Factor.Offset"=w411:dbl)
                n212 = call <vilib>:"svx_Oct_Waterfall XYZ Scale.vi"("Minimum"=w409, "Maximum"=w410, "Offset"=w411, "Multiplier"=w412) -> ("Scaled.Minimum"=w407:dbl, "Scaled.Maximum"=w408:dbl, "Range.Minimum"=w406:dbl, "Range.Maximum"=w405:dbl, "flipped?"=w413:bool)  [unwired: 3 in]
                n213 = property class="WFGraph (strict)"(reference=w414, "XScale.Flipped"=w413) -> ()  [unwired: 1 in, 2 out]
                n214 = Bundle By Name(cluster=w415, "X-Axis Range.Maximum"=w405, "X-Axis Range.Minimum"=w406, "X-Axis Range Scaled.Maximum"=w408, "X-Axis Range Scaled.Minimum"=w407) -> (w416:T1)
              }
              frame "Y-Axis" {
                n215 = Unbundle By Name(w427) -> ("Y-Axis Range Scaled.Maximum"=w418:dbl, "Y-Axis Scaling Factor.Multiplier"=w420:dbl, "Y-Axis Scaling Factor.Offset"=w419:dbl)
                n216 = call <vilib>:"svx_Oct_Waterfall XYZ Scale.vi"("Minimum"=w417, "Maximum"=w418, "Offset"=w419, "Multiplier"=w420) -> ("Scaled.Minimum"=w425:dbl, "Scaled.Maximum"=w424:dbl, "Range.Minimum"=w422:dbl, "Range.Maximum"=w423:dbl, "flipped?"=w421:bool)  [unwired: 3 in]
                n217 = property class="WFGraph (strict)"(reference=w426, "YScale.Flipped"=w421) -> ()  [unwired: 1 in, 2 out]
                n218 = Bundle By Name(cluster=w427, "Y-Axis Range.Maximum"=w423, "Y-Axis Range.Minimum"=w422, "Y-Axis Range Scaled.Maximum"=w424, "Y-Axis Range Scaled.Minimum"=w425) -> (w428:T1)
              }
              frame "Z-Axis" {
                n219 = Unbundle By Name(w437) -> ("Z-Axis Range Scaled.Maximum"=w429:dbl, "Z-Axis Scaling Factor.Multiplier"=w431:dbl, "Z-Axis Scaling Factor.Offset"=w430:dbl)
                n220 = call <vilib>:"svx_Oct_Waterfall XYZ Scale.vi"("Minimum"=w432, "Maximum"=w429, "Offset"=w430, "Multiplier"=w431) -> ("Scaled.Minimum"=w434:dbl, "Scaled.Maximum"=w436:dbl, "Range.Minimum"=w435:dbl, "Range.Maximum"=w433:dbl)  [unwired: 3 in, 1 out]
                n221 = Bundle By Name(cluster=w437, "Z-Axis Range.Maximum"=w433, "Z-Axis Range.Minimum"=w435, "Z-Axis Range Scaled.Maximum"=w436, "Z-Axis Range Scaled.Minimum"=w434) -> (w438:T1)
              }
            }
            n222 = Bundle By Name(cluster=w394, "Scales Changed"=TRUE) -> (w393:T6)
            n223 = local write "Range Maximum"(w392) -> ()
            n224 = local write "Range Minimum"(w391) -> ()
          }
          event "Range Maximum": Value Change {
            n225 = event-data() -> ("NewVal"=w450:dbl)  [unwired: 1 in]
            n226 = local read "Scale Axis"() -> (w447:enum16{"X-Axis", "Y-Axis", "Z-Axis"})
            n227 = Generate User Event(user event=w445, event data cluster=svx_Oct_Waterfall_Property_Page_User_Events."Update Graph" ("event data")) -> ()  [unwired: 2 in, 2 out]
            n228 = case shown="\"Z-Axis\"" w447 {
              tunnel: w452 -> [w463 w475 w485]
              tunnel: [w464 w476 w486] -> w451
              tunnel: w450 -> [w458 w470 w477]
              tunnel: w449 -> [w462 w474 _]
              tunnel: w448 -> [_ _ _]
              tunnel: w446 -> [_ _ _]
              tunnel: [w456 w468 w484] -> w440
              tunnel: [w455 w467 w483] -> w439
              frame "X-Axis" {
                n229 = Unbundle By Name(w463) -> ("X-Axis Range Scaled.Minimum"=w459:dbl, "X-Axis Scaling Factor.Multiplier"=w461:dbl, "X-Axis Scaling Factor.Offset"=w460:dbl)
                n230 = call <vilib>:"svx_Oct_Waterfall XYZ Scale.vi"("Minimum"=w459, "Maximum"=w458, "Offset"=w460, "Multiplier"=w461) -> ("Scaled.Minimum"=w455:dbl, "Scaled.Maximum"=w456:dbl, "Range.Minimum"=w453:dbl, "Range.Maximum"=w454:dbl, "flipped?"=w457:bool)  [unwired: 3 in]
                n231 = property class="WFGraph (strict)"(reference=w462, "XScale.Flipped"=w457) -> ()  [unwired: 1 in, 2 out]
                n232 = Bundle By Name(cluster=w463, "X-Axis Range.Maximum"=w454, "X-Axis Range.Minimum"=w453, "X-Axis Range Scaled.Maximum"=w456, "X-Axis Range Scaled.Minimum"=w455) -> (w464:T1)
              }
              frame "Y-Axis" {
                n233 = Unbundle By Name(w475) -> ("Y-Axis Range Scaled.Minimum"=w471:dbl, "Y-Axis Scaling Factor.Multiplier"=w473:dbl, "Y-Axis Scaling Factor.Offset"=w472:dbl)
                n234 = call <vilib>:"svx_Oct_Waterfall XYZ Scale.vi"("Minimum"=w471, "Maximum"=w470, "Offset"=w472, "Multiplier"=w473) -> ("Scaled.Minimum"=w467:dbl, "Scaled.Maximum"=w468:dbl, "Range.Minimum"=w465:dbl, "Range.Maximum"=w466:dbl, "flipped?"=w469:bool)  [unwired: 3 in]
                n235 = property class="WFGraph (strict)"(reference=w474, "YScale.Flipped"=w469) -> ()  [unwired: 1 in, 2 out]
                n236 = Bundle By Name(cluster=w475, "Y-Axis Range.Maximum"=w466, "Y-Axis Range.Minimum"=w465, "Y-Axis Range Scaled.Maximum"=w468, "Y-Axis Range Scaled.Minimum"=w467) -> (w476:T1)
              }
              frame "Z-Axis" {
                n237 = Unbundle By Name(w485) -> ("Z-Axis Range Scaled.Minimum"=w478:dbl, "Z-Axis Scaling Factor.Multiplier"=w480:dbl, "Z-Axis Scaling Factor.Offset"=w479:dbl)
                n238 = call <vilib>:"svx_Oct_Waterfall XYZ Scale.vi"("Minimum"=w478, "Maximum"=w477, "Offset"=w479, "Multiplier"=w480) -> ("Scaled.Minimum"=w483:dbl, "Scaled.Maximum"=w484:dbl, "Range.Minimum"=w482:dbl, "Range.Maximum"=w481:dbl)  [unwired: 3 in, 1 out]
                n239 = Bundle By Name(cluster=w485, "Z-Axis Range.Maximum"=w481, "Z-Axis Range.Minimum"=w482, "Z-Axis Range Scaled.Maximum"=w484, "Z-Axis Range Scaled.Minimum"=w483) -> (w486:T1)
              }
            }
            n240 = Bundle By Name(cluster=w442, "Scales Changed"=TRUE) -> (w441:T6)
            n241 = local write "Range Maximum"(w440) -> ()
            n242 = local write "Range Minimum"(w439) -> ()
          }
          event "Autoscale": Value Change {
            n243 = event-data() -> ("NewVal"=w491:bool)  [unwired: 1 in]
            n244 = Generate User Event(user event=w496, event data cluster=svx_Oct_Waterfall_Property_Page_User_Events."Update Graph" ("event data")) -> ()  [unwired: 2 in, 2 out]
            n245 = local read "Scale Axis"() -> (w487:enum16{"X-Axis", "Y-Axis", "Z-Axis"})
            n246 = Select(t=u8 2, s=w491, f=u8 0 ("Disabled")) -> (s? t:f=w490:u8)
            n247 = case shown="\"X-Axis\"" w487 {
              tunnel: w498 -> [w501 w504 w507]
              tunnel: [w500 w503 w506] -> w497
              tunnel: w490 -> [w499 w502 w505]
              frame "X-Axis" {
                n248 = Bundle By Name(cluster=w501, "AutoScale X"=w499) -> (w500:T1)
              }
              frame "Y-Axis" {
                n249 = Bundle By Name(cluster=w504, "AutoScale Y"=w502) -> (w503:T1)
              }
              frame "Z-Axis" {
                n250 = Bundle By Name(cluster=w507, "AutoScale Z"=w505) -> (w506:T1)
              }
            }
            n251 = Bundle By Name(cluster=w493, "Scales Changed"=TRUE) -> (w492:T6)
            n252 = property on="Range Minimum" class="DigNum (strict)"("Disabled"=w490) -> ()  [unwired: 2 in, 2 out]
            n253 = property on="Range Maximum" class="DigNum (strict)"("Disabled"=w490) -> ()  [unwired: 2 in, 2 out]
          }
          event "FP Axis": Value Change {
            n254 = event-data() -> ("NewVal"=w515:enum16{"X-Axis", "Y-Axis", "Z-Axis"})  [unwired: 1 in]
            n255 = case shown="\"X-Axis\", Default" w515 {
              tunnel: w513 -> [w517 w519 w521]
              tunnel: [w516 w518 w520] -> w508
              frame "X-Axis", Default {
                n256 = Unbundle By Name(w517) -> ("X-Scale Format Str"=w516:string)
              }
              frame "Y-Axis" {
                n257 = Unbundle By Name(w519) -> ("Y-Scale Format Str"=w518:string)
              }
              frame "Z-Axis" {
                n258 = Unbundle By Name(w521) -> ("Z-Scale Format Str"=w520:string)
              }
            }
            n259 = call <vilib>:"svx_Oct_Parse Format String.vi"("Format string"=w508) -> ("trailing zeros"=w509:bool, "Precision Type"=w510:u16, "Digits"=w511:u8, "Type"=w512:i32)  [unwired: 6 in, 1 out]
            n260 = local write "Precision Type"(w510) -> ()
            n261 = local write "Type"(w512) -> ()
            n262 = local write "trailing zeros"(w509) -> ()
            n263 = local write "Digits"(w511) -> ()
          }
          event "Type", "Precision Type", "Digits", "trailing zeros": Value Change {
            n264 = event-data() -> ()  [unwired: 1 in, 1 out]
            n265 = call <vilib>:"svx_Oct_Build Format String.vi"("trailing zeros"="trailing zeros", "Precision Type"="Precision Type", "Digits"="Digits", "Type"="Type") -> ("String"=w528:string)
            n266 = case shown="\"X-Axis\"" "FP Axis" {
              tunnel: w534 -> [w538 w542 w546]
              tunnel: [w537 w541 w545] -> w533
              tunnel: w528 -> [w536 w539 w544]
              tunnel: w527 -> [w535 w540 _]
              tunnel: w526 -> [_ _ w543]
              frame "X-Axis" {
                n267 = Bundle By Name(cluster=w538, "X-Scale Format Str"=w536) -> (w537:T1)
                n268 = property class="WFGraph (strict)"(reference=w535, "XScale.FormatString"=w536) -> ()  [unwired: 1 in, 2 out]
              }
              frame "Y-Axis" {
                n269 = Bundle By Name(cluster=w542, "Y-Scale Format Str"=w539) -> (w541:T1)
                n270 = property class="WFGraph (strict)"(reference=w540, "YScale.FormatString"=w539) -> ()  [unwired: 1 in, 2 out]
              }
              frame "Z-Axis" {
                n271 = Bundle By Name(cluster=w546, "Z-Scale Format Str"=w544) -> (w545:T1)
                n272 = property class="WFGraph (strict)"(reference=w543, "YScale.FormatString"=w544) -> ()  [unwired: 1 in, 2 out]
              }
            }
            n273 = Bundle By Name(cluster=w531, "Scales Changed"=TRUE) -> (w530:T6)
          }
          event "OK": Value Change {
            w547 = FALSE
            n274 = event-data() -> ()  [unwired: 1 in, 1 out]
            n275 = Generate User Event(user event=w548, event data cluster=svx_Oct_Waterfall_Property_Page_User_Events."Exit" ("Property Page User Events")) -> ()  [unwired: 2 in, 2 out]
            n276 = local write "Cancel?"(w547) -> ()
          }
          event "Cancel": Value Change; Panel Close {
            n277 = event-data() -> ()  [unwired: 1 in, 1 out]
            n278 = stacked-sequence {
              tunnel: w560 -> [w564 w582 w600 _]
              tunnel: w559 -> [w562 _ _ _]
              tunnel: w558 -> [_ w580 _ w628]
              tunnel: w557 -> [_ w579 w596 _]
              tunnel: w556 -> [_ _ _ _]
              tunnel: w555 -> [_ w578 _ _]
              tunnel: w554 -> [w561 _ _ _]
              tunnel: w553 -> [_ _ w598 _]
              tunnel: w552 -> [_ _ w597 _]
              frame #0 {
                n279 = Unbundle By Name(w564) -> ("Container Changed"=w563:bool)
                n280 = case shown="True" w563 {
                  tunnel: w562 -> [_ w573]
                  tunnel: w561 -> [_ w565]
                  frame False {
                  }
                  frame True {
                    n281 = Unbundle(w565) -> ("Label.Text"=w572:string, "Label.Visible"=w571:bool, "Caption.Text"=w570:string, "Caption.Visible"=w569:bool, "Disabled"=w568:u8, "Desc"=w567:string, "TipStrip"=w566:string)
                    n282 = property class="Ctl"(reference=w573, "Label.Text"=w572, "Label.Visible"=w571, "Caption.Text"=w570, "Caption.Visible"=w569, "Disabled"=w568, "Desc"=w567, "TipStrip"=w566) -> ()  [unwired: 1 in, 2 out]
                  }
                }
              }
              frame #1 {
                n283 = Unbundle By Name(w582) -> ("Waveform Changed"=w581:bool)
                n284 = local read "# Plots Updated in"() -> (w574:i32)
                n285 = Unbundle By Name(w579) -> ("Plot Transparency"=w575:bool, "Background Color"=w577:u32, "Plot Color"=w576:u32)
                n286 = case shown="True" w581 {
                  tunnel: w580 -> [_ w591]
                  tunnel: w578 -> [_ w583]
                  tunnel: w577 -> [_ w584]
                  tunnel: w576 -> [_ w589]
                  tunnel: w575 -> [_ w588]
                  tunnel: w574 -> [_ w585]
                  frame False {
                  }
                  frame True {
                    n287 = Select(t=u32 16777216, s=w588, f=w584) -> (s? t:f=w586:u32)
                    n288 = for {
                      N: w585 -> [_]
                      tunnel: w583 -> [w594]
                      tunnel: w586 -> [w592]
                      tunnel: w589 -> [w593]
                      i -> [w595]
                      n289 = property class="XYGraph (strict)"(reference=w594, "Active Plot"=w595, "Plot.Fill/Pt. Color"=w592, "Plot.Plot Color"=w593) -> ()  [unwired: 1 in, 2 out]
                    }
                    n290 = property class="XYGraph (strict)"(reference=w583, "BG Color"=w584) -> ()  [unwired: 1 in, 2 out]
                    n291 = Generate User Event(user event=w591, event data cluster=svx_Oct_Waterfall_Property_Page_User_Events."Redraw Frame" ("Property Page User Events")) -> ()  [unwired: 2 in, 2 out]
                  }
                }
              }
              frame #2 {
                n292 = Unbundle By Name(w600) -> ("Scales Changed"=w599:bool)
                n293 = case shown="True" w599 {
                  tunnel: w598 -> [_ w614]
                  tunnel: w597 -> [_ w618]
                  tunnel: w596 -> [_ w625]
                  frame False {
                  }
                  frame True {
                    n294 = Unbundle By Name(w625) -> ("X-Axis Scaling Factor.Multiplier"=w613:dbl, "Y-Axis Scaling Factor.Multiplier"=w611:dbl, "X-Axis Range Scaled.Minimum"=w624:dbl, "X-Axis Range Scaled.Maximum"=w623:dbl, "X-Axis Name"=w622:string, "Y-Axis Range Scaled.Minimum"=w621:dbl, "Y-Axis Range Scaled.Maximum"=w620:dbl, "Y-Axis Name"=w619:string, "X-Scale Visible"=w608:bool, "Y-Scale Visible"=w609:bool, "X-Scale Label Visible"=w605:bool, "Y-Scale Label Visible"=w606:bool, "X-Scale Format Str"=w603:string, "Y-Scale Format Str"=w602:string, "Z-Axis Range Scaled.Minimum"=w617:dbl, "Z-Axis Range Scaled.Maximum"=w616:dbl, "Z-Axis Name"=w615:string, "Z-Scale Visible"=w607:bool, "Z-Scale Label Visible"=w604:bool, "Z-Scale Format Str"=w601:string)
                    n295 = Less Than 0?(x=w613) -> (x < 0?=w612:bool)
                    n296 = Less Than 0?(x=w611) -> (x < 0?=w610:bool)
                    n297 = property class="WFGraph (strict)"(reference=w614, "XScale.Flipped"=w612, "YScale.Flipped"=w610, "XScale.Minimum"=w624, "XScale.Maximum"=w623, "XScale.NameLbl.Text"=w622, "YScale.Minimum"=w621, "YScale.Maximum"=w620, "YScale.NameLbl.Text"=w619, "XScale.Visible"=w608, "YScale.Visible"=w609, "XScale.NameLbl.Visible"=w605, "YScale.NameLbl.Visible"=w606, "XScale.FormatString"=w603, "YScale.FormatString"=w602) -> ()  [unwired: 1 in, 2 out]
                    n298 = property class="WFGraph (strict)"(reference=w618, "YScale.Minimum"=w617, "YScale.Maximum"=w616, "YScale.NameLbl.Text"=w615, "YScale.Visible"=w607, "YScale.NameLbl.Visible"=w604, "YScale.FormatString"=w601) -> ()  [unwired: 1 in, 2 out]
                  }
                }
              }
              frame #3 {
                n299 = Generate User Event(user event=w628, event data cluster=svx_Oct_Waterfall_Property_Page_User_Events."Exit" ("Property Page User Events")) -> ()  [unwired: 2 in, 2 out]
                "Cancel?" <- "Cancel"
              }
            }
          }
          event "Help": Value Change {
            n300 = event-data() -> ()  [unwired: 1 in, 1 out]
            n301 = Control Online Help(2:path "<helpdir>/sndvibtk.chm" ("Path to the help file"), 3:"Octave_Waterfall_Graph_DB.html" ("String to search for"), 4:enum16{"Contents", "Key", "Close"}."Key" ("Operation")) -> ()  [unwired: 1 in, 1 out]
          }
          event User Event {
            n302 = event-data() -> ("Property Page User Events"=w642:T5)  [unwired: 1 in]
            n303 = case shown="\"Redraw Frame\", Default" w642 {
              tunnel: [_ _ TRUE] -> w641
              tunnel: w640 -> [w673 w710 _]
              tunnel: w639 -> [w672 w701 _]
              tunnel: w638 -> [_ w705 _]
              tunnel: w637 -> [w669 w703 w722]
              tunnel: w636 -> [_ _ w723]
              tunnel: w635 -> [_ w696 _]
              tunnel: [w669 w693 w722] -> w634
              frame "Redraw Frame", Default {
                w644 = cluster{"x":i16, "y":i16} {"x"=0, "y"=0} ("cluster")
                w654 = u32 0 ("Offset")
                w675 = T8 {"Width"=1, "Style"=enum."Solid"} ("pen")
                n304 = property class="WFGraph (strict)"(reference=w672) -> ("Width"=w649:u32, "Height"=w650:u32)  [unwired: 1 in, 2 out]
                n305 = property class="XYGraph (strict)"(reference=w673) -> (reference out=w671:refnum<vi>, "Width"=w647:u32, "Height"=w648:u32)  [unwired: 1 in, 1 out]
                n306 = Unbundle By Name(w669) -> ("Frame Color"=w670:u32)
                n307 = Subtract(x=w647, y=w649) -> (x-y=w658:u32)
                n308 = Subtract(x=w648, y=w650) -> (x-y=w651:u32)
                n309 = Increment(x=w647) -> (x+1=w652:u32)
                n310 = Decrement(x=w650) -> (x-1=w659:u32)
                n311 = Increment(x=w658) -> (x+1=w657:u32)
                n312 = Decrement(x=w654) -> (x-1=w655:u32)
                n313 = Decrement(x=w651) -> (x-1=w656:u32)
                n314 = Increment(x=w654) -> (x+1=w653:u32)
                n315 = Decrement(x=w648) -> (x-1=w662:u32)
                n316 = Increment(x=w649) -> (x+1=w661:u32)
                n317 = Decrement(x=w648) -> (x-1=w660:u32)
                n318 = Bundle(cluster=w644, "x"=w652, "y"=w659) -> (w663:cluster{"x":i16, "y":i16})
                n319 = Bundle(cluster=w644, "x"=w657, "y"=w659) -> (w664:cluster{"x":i16, "y":i16})
                n320 = Bundle(cluster=w644, "x"=w657, "y"=w655) -> (w668:cluster{"x":i16, "y":i16})
                n321 = Bundle(cluster=w644, "x"=w653, "y"=w656) -> (w667:cluster{"x":i16, "y":i16})
                n322 = Bundle(cluster=w644, "x"=w653, "y"=w662) -> (w665:cluster{"x":i16, "y":i16})
                n323 = Bundle(cluster=w644, "x"=w661, "y"=w660) -> (w666:cluster{"x":i16, "y":i16})
                n324 = Build Array(w663, w664, w668, w667, w665, w664) -> (w646:cluster{"x":i16, "y":i16}[])
                n325 = Build Array(w665, w666, w663) -> (w645:cluster{"x":i16, "y":i16}[])
                n326 = call <vilib>:"Draw Multiple Lines.vi"("line endpoints"=w646, "color(black)"=w670, "pen"=w675) -> ("new picture"=w674:picture)  [unwired: 6 in]
                n327 = call <vilib>:"Draw Multiple Lines.vi"("line endpoints"=w645, "color(black)"=w670, "pen"=w675) -> ("new picture"=w676:picture)  [unwired: 6 in]
                n328 = property on="Property Node" class="XYGraph (strict)"(reference=w671, "PlotImages.Back"=w674, "PlotImages.Front"=w676) -> ()  [unwired: 1 in, 2 out]
              }
              frame "Update Graph" {
                # "see if Z scale\nshould be flipped"
                n329 = call <vilib>:"svx_Oct_Autoscale Ranges.vi"("Display State In"=w703, "Data Array In"=w705) -> ("Cropped Info out"=w679:cluster{"First Index":i32, "Length":i32}, "Display State Out"=w702:T1, "Data Array Out"=w711:T2)  [unwired: 5 in, 2 out]
                n330 = local read "Scale Axis"() -> (w704:enum16{"X-Axis", "Y-Axis", "Z-Axis"})
                n331 = call <vilib>:"svx_Oct_Fit Data to Scale.vi"("Cropped Info"=w679, "Display State In"=w702, "Data In"=w711) -> ("Waveform YScale Max"=w707:dbl, "Waveform XScale Max"=w708:dbl, "Display State Out"=w693:T1, "Data Out"=w706:T2, "Markers"=w688:dbl[])  [unwired: 4 in]
                n332 = Unbundle By Name(w693) -> ("X-Axis Range Scaled.Minimum"=w700:dbl, "X-Axis Range Scaled.Maximum"=w699:dbl, "Y-Axis Range Scaled.Minimum"=w698:dbl, "Y-Axis Range Scaled.Maximum"=w697:dbl, "Z-Axis Range Scaled.Minimum"=w695:dbl, "Z-Axis Range Scaled.Maximum"=w694:dbl, "Rev Z Order"=w684:bool, "Z-Axis Scaling Factor.Multiplier"=w683:dbl)
                n333 = case shown="\"X-Axis\"" w704 {
                  tunnel: [w714 w717 w720] -> w692
                  tunnel: [w713 w716 w719] -> w691
                  tunnel: w693 -> [w712 w715 w718]
                  frame "X-Axis" {
                    n334 = Unbundle By Name(w712) -> ("X-Axis Range Scaled.Minimum"=w714:dbl, "X-Axis Range Scaled.Maximum"=w713:dbl)
                  }
                  frame "Y-Axis" {
                    n335 = Unbundle By Name(w715) -> ("Y-Axis Range Scaled.Minimum"=w717:dbl, "Y-Axis Range Scaled.Maximum"=w716:dbl)
                  }
                  frame "Z-Axis" {
                    n336 = Unbundle By Name(w718) -> ("Z-Axis Range Scaled.Minimum"=w720:dbl, "Z-Axis Range Scaled.Maximum"=w719:dbl)
                  }
                }
                n337 = Unbundle By Name(w693) -> ("X-Axis Range.Minimum"=w678:dbl, "Y-Axis Range.Minimum"=w709:dbl)
                n338 = Unbundle By Name(w706) -> ("Plots"=w680:cluster{"X":dbl[], "Y":dbl[]}[], "dz"=w682:dbl)
                n339 = Less Than 0?(x=w683) -> (x < 0?=w687:bool)
                n340 = Less Than 0?(x=w682) -> (x < 0?=w686:bool)
                n341 = Logarithm Base 10(1:w678) -> (0:w677:dbl)
                n342 = Exclusive Or(1:w686, 2:w687) -> (0:w685:bool)
                n343 = property on="Property Node" class="WFGraph (strict)"(reference=w701, "XScale.Minimum"=w700, "XScale.Maximum"=w699, "YScale.Minimum"=w698, "YScale.Maximum"=w697) -> ()  [unwired: 1 in, 2 out]
                n344 = property on="Property Node" class="XYGraph (strict)"(reference=w710, "XScale.Minimum"=w677, "YScale.Minimum"=w709, "XScale.Maximum"=w708, "YScale.Maximum"=w707, "Value"=w680) -> ()  [unwired: 1 in, 2 out]
                n345 = Exclusive Or(1:w684, 2:w685) -> (0:w681:bool)
                n346 = property on="Property Node" class="WFGraph (strict)"(reference=w696, "YScale.Flipped"=w681, "YScale.Minimum"=w695, "YScale.Maximum"=w694, "YScale.MarkerVals[]"=w688) -> ()  [unwired: 1 in, 2 out]
                n347 = Max & Min(x=w692, y=w691) -> (max(x,y)=w690:dbl, min(x,y)=w689:dbl)
                n348 = local write "Range Maximum"(w690) -> ()
                n349 = local write "Range Minimum"(w689) -> ()
              }
              frame "Exit" {
                n350 = Destroy User Event(user event=w723) -> ()  [unwired: 1 in, 1 out]
                "# Plots Updated out" <- "# Plots Updated in"
              }
            }
          }
        }
      }
    }
  }
  "State out" <- w5
